vi "Configuração.vi"() -> ()   [LabVIEW 2018]
uses:
  Global_Telescopio.vi
panel:
  in  "URL do finals2000A.all:":string
  in  "Case Constant\n(See Context Help) 4":bool
  in  "Case Constant\n(See Context Help)":bool
  out "error out":errorcluster
  in  "Geral":T1(tab)=enum."Pos. Cúpula"
  in  "wheather timeout":bool
  in  "Tempo sem dados":dbl=120.0 caption="segundos" min=0.0
  in  "PressãoMax":dbl=1200.0 caption="mbar"
  in  "UmidadeMax":dbl=100.0 caption="%"
  in  "TemperaturaMax":dbl=30.0 caption="ºC"
  in  "PressãoMin":dbl=500.0 caption="mbar"
  in  "UmidadeMin":dbl caption="%"
  in  "TemperaturaMin":dbl caption="ºC"
  in  "Salvar valores":bool
  in  "Pressão atmosférica":dbl=880.0 caption="mbar"
  in  "Umidade":dbl=88.0 caption="%"
  in  "Temperatura":dbl=15.0 caption="ºC"
  in  "Default Met":bool
  in  "Memorizar Default Met":bool
  in  "Caminho Estação Meteorológica":string="V 1.0.0 arquivo obsoleto. Usado apenas PUB ZeroMQ."
  in  "Desloc_Min_Cúpula":i32=2 min=2
  in  "OffsetCupula":dbl=135.0 format="%#_11g"
  in  "Salvar dados cupula":bool
  in  "OffsetZ":dbl=-0.28 format="%#_11g"
  in  "OffsetY":dbl format="%#_11g"
  in  "OffsetX":dbl format="%#_11g"
  in  "DistEixos":dbl=-0.62 format="%#_11g"
  in  "RaioCup":dbl=3.2 format="%#_11g"
  in  "LATrad":dbl=5.889885056 format="%#_11g"
  out "Calagem DEC":string
  out "Calagem AH":string
  in  "LoadCalagem":bool
  in  "Instrumento":u16(ring) items=["Coude A+", "Coude B+", "ECass+", "Eucalyptus+", "Cam 1+", "Cam 2*", "Cam4 + IV*", "Polarimetro*", "Fortrap*", "Cam1 RF*", "Coude C+", "MUSICOS*", "+Já testado", "* nao config", "cam 1 s/rf", "cam1srf/luca+focali", "Coude A/luca", "ECass/luca", "Cam1+rf+luca", "MUSICOS+Luca", "Camiv+Luca", "Cam2+Luca", "Cam1+rf+luca+Ixon", "Cam1+rf+luca+Ikon", "CoudeTeste"]
  in  "Conf. Instrumentos":bool
  in  "Tabela Instrumentos":string[][](table)=[["Coude", "281.52", " 11.53", "S", "S", "0.462", "23.1", "23.1"], ["Cassegrain", "281.52", " 11.53", "S", "S", "0.462", "23.1", "23.1"], ["Eucalyptus", "281.52", " 11.53", "S", "S", "0.462", "23.1", "23.1"], ["Cam 1", "281.52", " 11.53", "S", "S", "0.462", "23.1", "23.1"], ["Cam 2", "281.52", " 11.53", "S", "S", "0.462", "23.1", "23.1"], ["Cam IV", "281.52", " 11.53", "S", "S", "0.462", "23.1", "23.1"], ["Polarimetro", "281.52", " 11.53", "S", "S", "0.462", "23.1", "23.1"], ["Fortrap", "281.52", " 11.53", "S", "S", "0.462", "23.1", "23.1"]]
  in  "CorrecaoMin":dbl=0.1
  in  "tel_sts1":bool[](array[boolean])=[TRUE, TRUE, TRUE, TRUE, FALSE, FALSE, TRUE]
  in  "Senha LEAF":string
  in  "Enable ventilador":bool=TRUE
  in  "habilita supervisao":bool
  in  "Tempo delay":i32=1
  in  "Limite Oeste":dbl=5.0 min=-12.0 max=12.0 step=0.1
  in  "Limite Leste":dbl=-4.5 min=-12.0 max=12.0 step=0.1
  out "DownloadWait":bool
  out "DownloadOK":bool caption="OK"
  in  "Download_Finals2000A.all":bool
  in  "Tempo Atualização All Sky":i32=1 min=1
  in  "Tempo Atualização Cam 3":i32=1 min=1
  in  "Tempo Atualização Cam 2":i32=1 min=1
  in  "Tempo Atualização Cam 1":i32=1 min=1
  in  "Tempo Atualização Cam 0":i32=1 min=1
  out "Ângulo Zenital":dbl format="%#.1f"
  out "Azimute":dbl format="%#.1f"
  in  "Tabela Proteção":string[][](table)=[["0", "360", "70", "60", "65"]]
  in  "Raio Máximo":dbl=5.0 min=0.0 max=90.0 step=0.1
  in  "Z_Max":dbl
  in  "Z_Libera":dbl
  in  "Z_Segurança":dbl
  in  "Hour Angle":string="00 00 0,00" caption="Dest AH"
  in  "Dest Dec":string="00 00 00,00"
  in  "SALVA CONFIG":bool
  out "DestDEC":dbl
  in  "DestCUP":i32
  out "DestAH":dbl
  in  "Caminho camera":string
  in  "Hora vent inicial":i32=1 min=0 max=86399 step=1 format="%<%H:%M:%S>t"
  in  "Hora vent final":i32=1 min=0 max=86399 step=1 format="%<%H:%M:%S>t"
  in  "ENGENHARIA":bool
  # "Configuração do Sistema"
  # "Caminho completo da Estação Meteorológica\nEx: http://200.131.64.185/clima/download.txt"
  # "Especifica o tempo para sinalizar que o TCSPD não está\nrecebendo os dados da estação meteorológica."
  # "Usar valores default se ocorrer a sinalização descrita acima."
  # "Valores Médios"
  # "Limite Mínimo"
  # "Limite Máximo"
  # "Quando \"Default Met\" for selecionado, sempre serão usados os valores médios (default) de temperatura, umidade e pressão atmosférica no cálculo da refração atmostérica e não os valores lidos da estação meteorológica, mesmo que estes sejam válidos e corretos."
  # "Se alguma leitura da estação meteorológica estiver fora dos limites acima, aquele valor será automaticamente substituído pelo seu valor médio."
  # "CONSTANTES DA CÚPULA"
  # "1,60m"
  # "IAG"
  # "5,889885056"
  # "5,889885056"
  # "7,525"
  # "3,20"
  # "-0,62"
  # "1,570"
  # "0,000"
  # "0,000"
  # "0,000"
  # "0,000"
  # "0,300"
  # "-0,28"
  # "136,0"
  # "-135,0"
  # "4"
  # "2"
  # "Valores default para o IAG (03/03/2011)"
  # "Ao precionar as Teclas de Captura\né necessário selecionar  a Região \nde interesse da imagem!"
  # "Selecione a Captrua\na ser posicionada"
  # "Seriais\nAuto Guider"
  # "Ângulo\nRotator"
  # "Ângulo\nNorte"
  # "Img.\nEsp."
  # "No\nCass."
  # "Escala\nPlaca"
  # "Calagem\nAH (\")"
  # "Calagem\nDEC (\")"
  # "Posição\nFoco"
  # "Escolha do Instrumento"
  # "Instrumento"
  # "Calagem"
  # "Carrega a calagem do telescópio com a calagem inicial do instrumento"
  # "CorrecaoMin: Valor em arcsec utilizado como limite para mover os\neixos AH e DEC nos processos de guiagem automática (auto-guider)\ne de offset do sistema de aquisição. Não será executado nenhum \nmovimento desses processos com deslocamento inferior a CorrecaoMin."
  # "Parâmetros PARK"
  # "Radianos"
  # "-->"
  # "Faixa do Azimute\n   De:              Ate:"
  # "Ângulo Zenital\n  Máx:       Segur.:       Libera:"
  # "-->"
  # "Raio da Calagem Local"
  # "Graus"
  # "Tempo de delay de comunicação"
  # "Arquivo finals2000A.all para precessão"
  # "Habilita Supervisão do Controlador"
  # "Horas"
  # "Horas"
  # "C:\\TCS\\ARQUIVOS\\finals2000A.all,  2,2Mb"
  # "Ventilador"
  # "Endereço da câmera"
  # "Usada na janela popup do Leaf e na\naba DOME que tem dupla função:abrir trapeira e habilitar movimento do telescópio com plataforma alta."
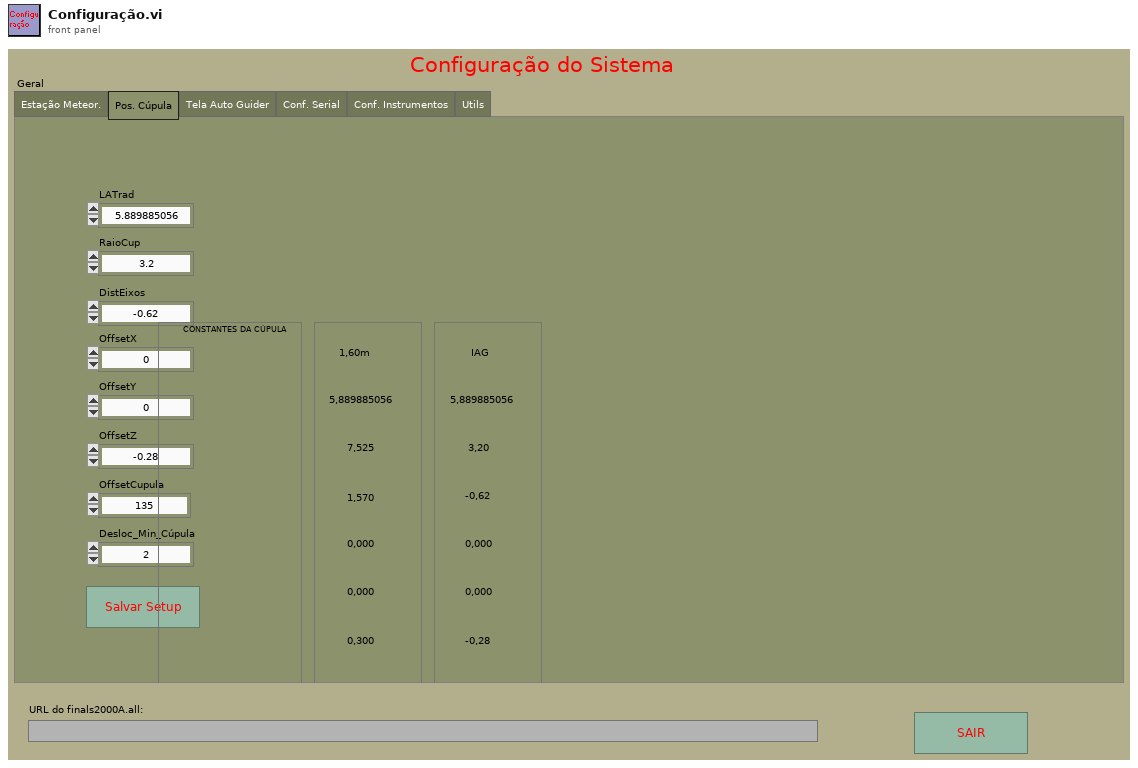
[diagram p1: front panel]
types:
  T1 = enum32{"Estação Meteor.", "Pos. Cúpula", "Tela Auto Guider", "Conf. Serial", "Conf. Instrumentos", "Utils"}
  T2 = cluster{"temperatura":dbl, "umidade":dbl, "pressao":dbl, "temperaturaMin":dbl, "umidadeMin":dbl, "pressaoMin":dbl, "temperaturaMax":dbl, "umidadeMax":dbl, "pressaoMax":dbl, "tempoSemDados":dbl}
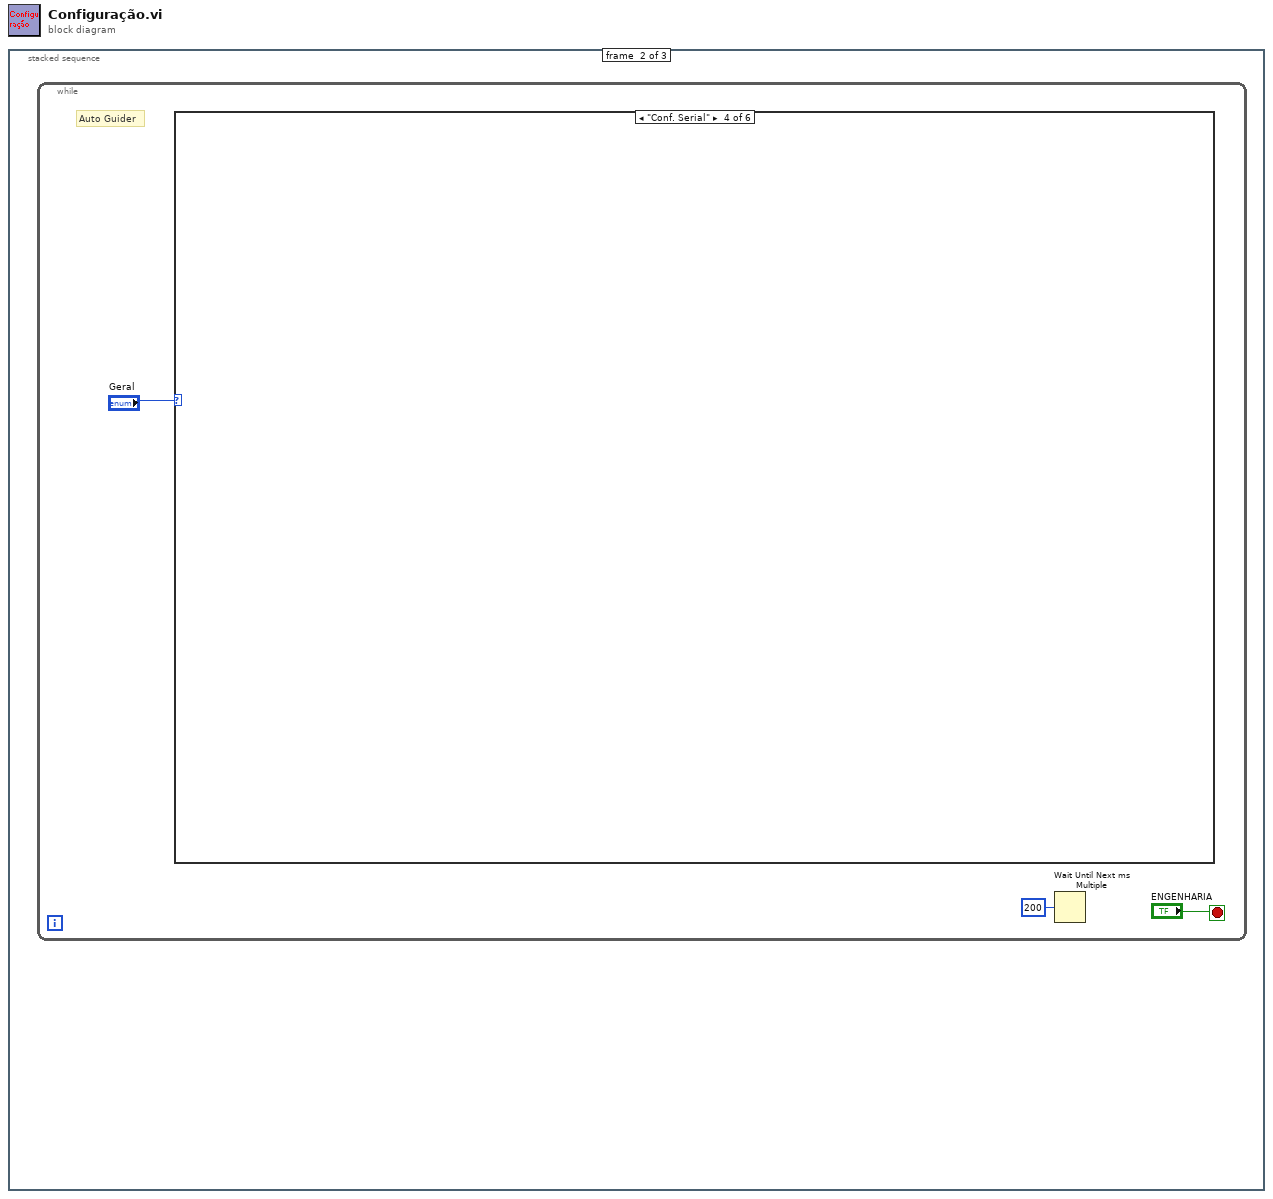
[diagram p0: block diagram]
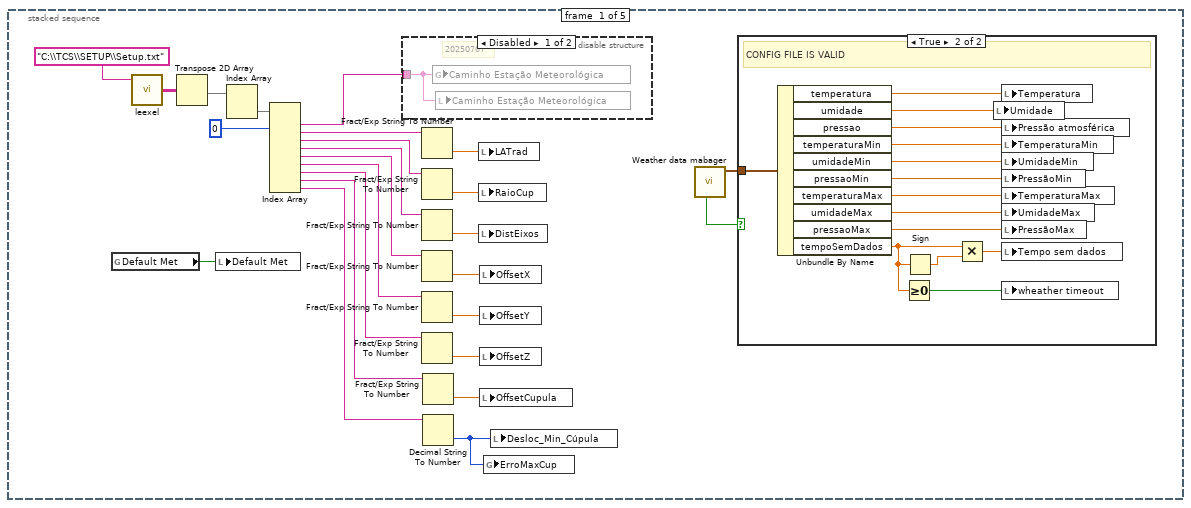
[diagram p3: hidden frame]
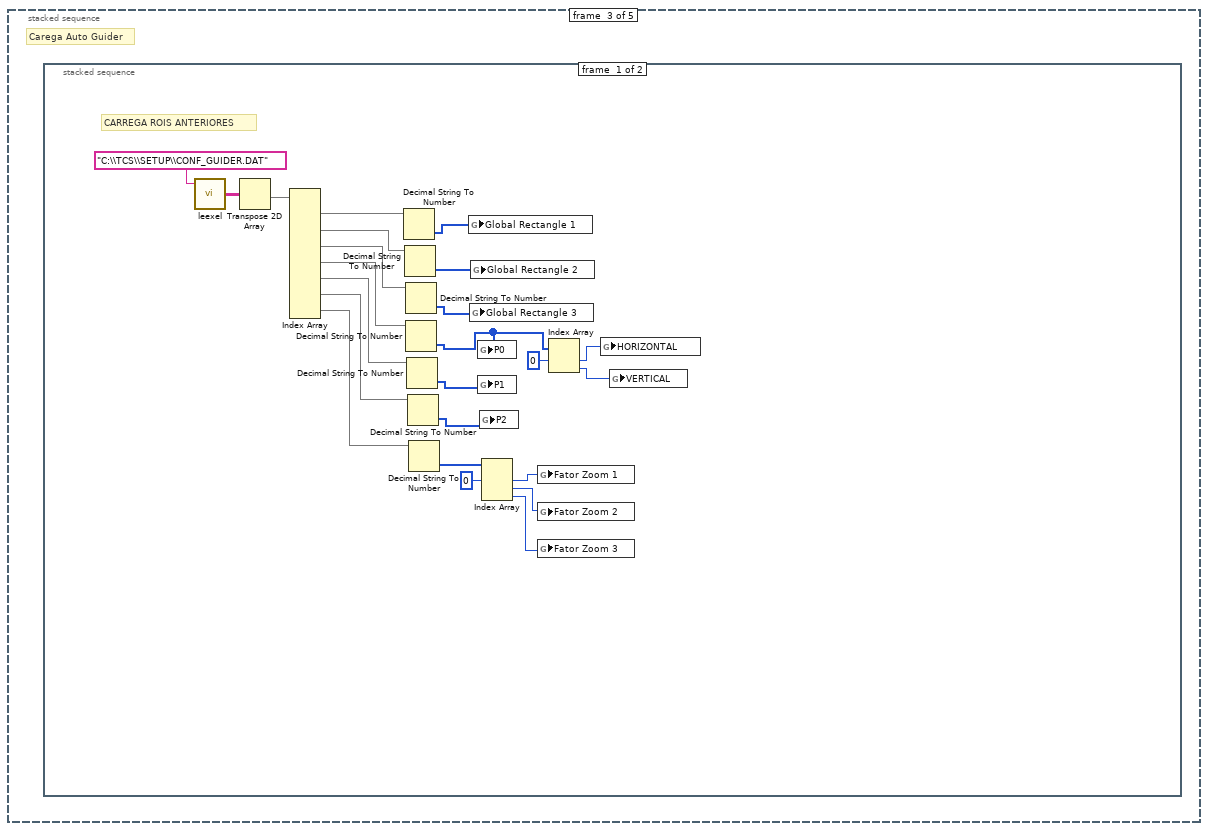
[diagram p6: hidden frame]
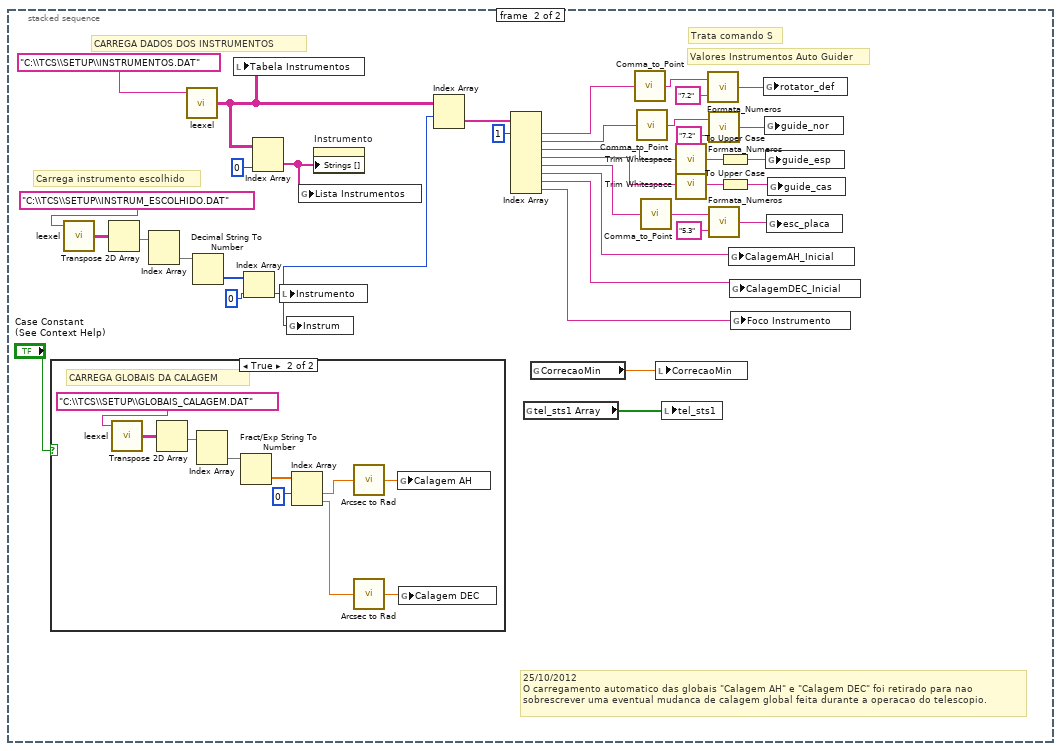
[diagram p7: hidden frame]
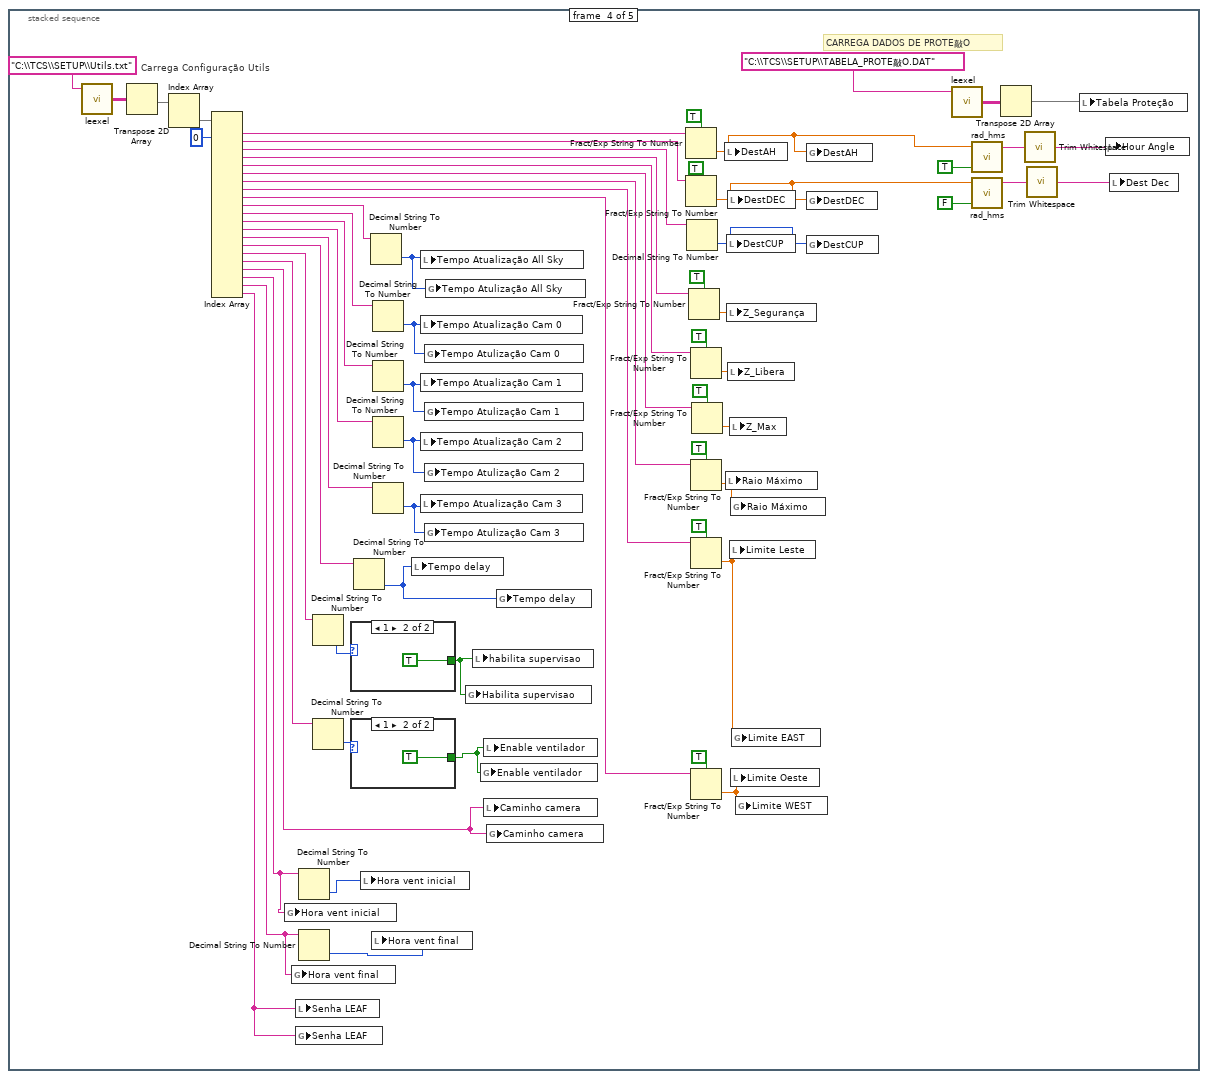
[diagram p9: hidden frame]
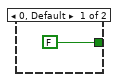
[diagram p10: hidden frame]
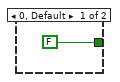
[diagram p11: hidden frame]
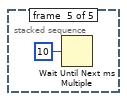
[diagram p12: hidden frame]
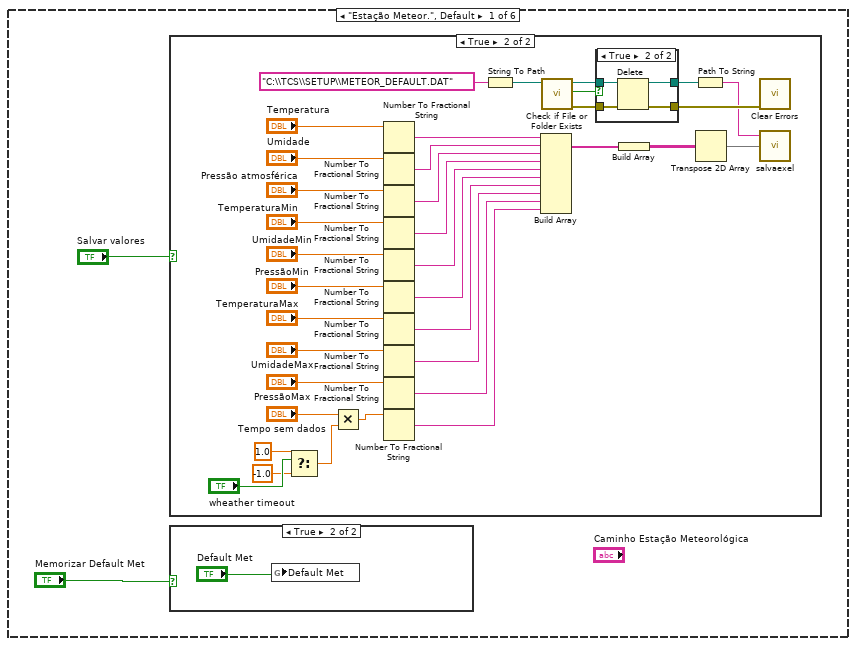
[diagram p13: hidden frame]
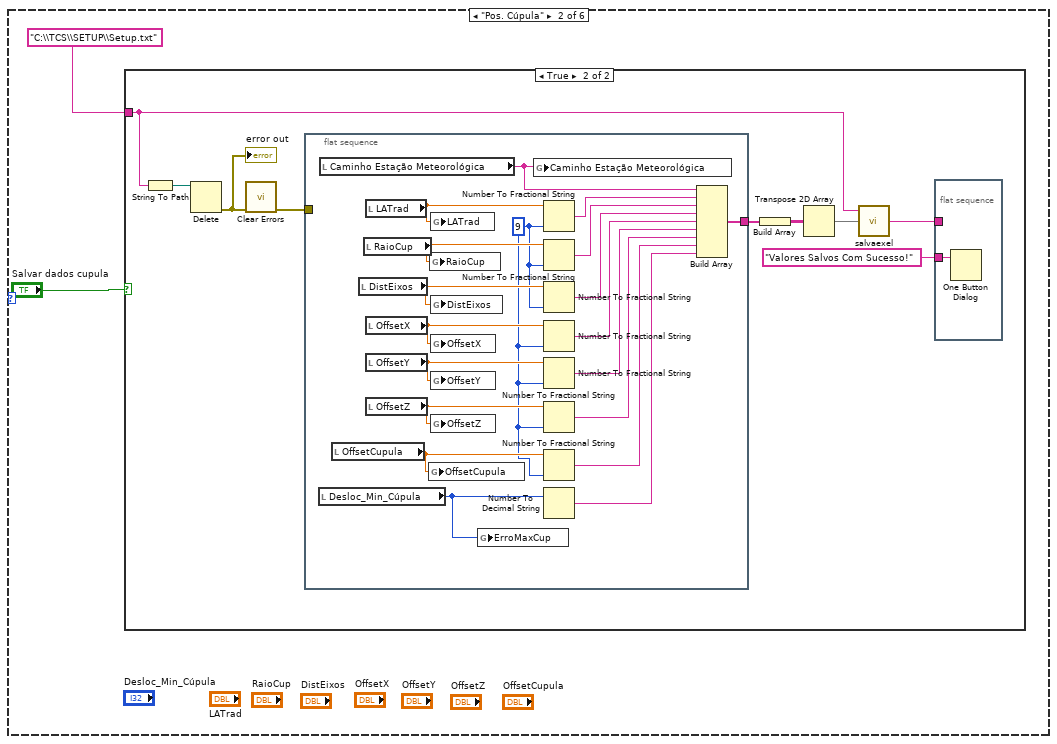
[diagram p17: hidden frame]
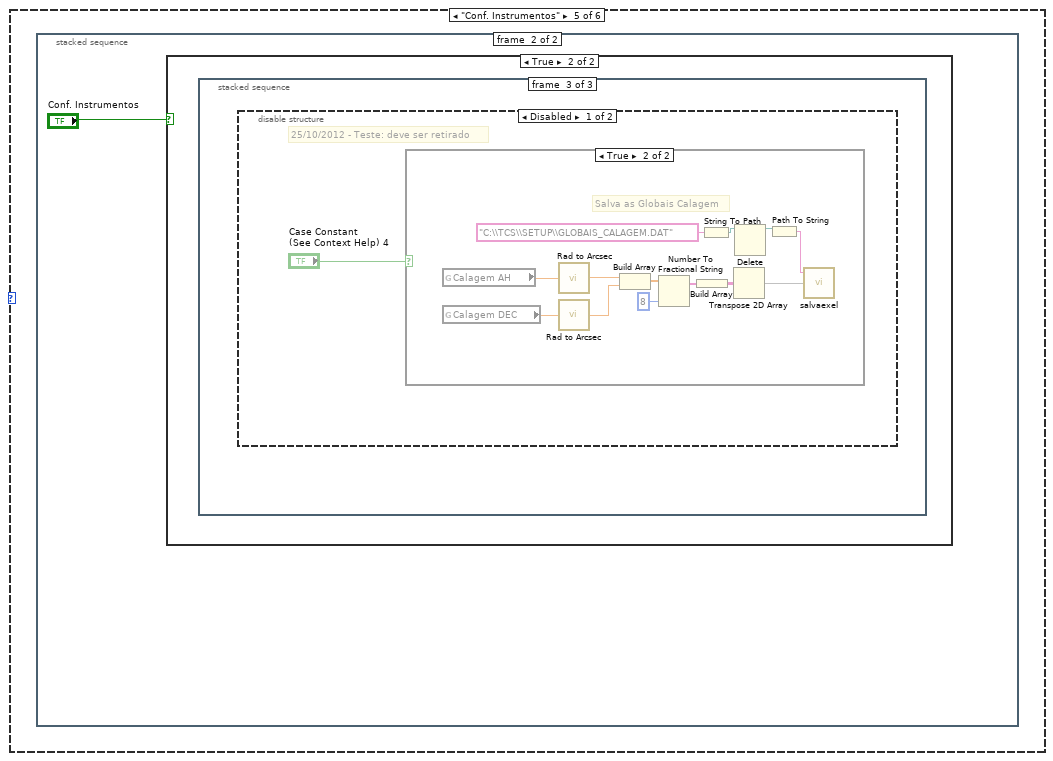
[diagram p20: hidden frame]
diagram:
  n1 = stacked-sequence {
    frame #0 {
      n2 = stacked-sequence {
        frame #0 {
          n3 = global read "Global_Telescopio.vi" "Default Met"() -> (w3:bool)
          n4 = call "leexel.vi"("path"="C:\\TCS\\SETUP\\Setup.txt") -> ("array 5"=w24:string[][])  [unwired: 4 in]
          n5 = Transpose 2D Array(2D array=w24) -> (transposed array=w23:string[][])
          n6 = local write "Default Met"(w3) -> ()
          n7 = Index Array(array=w23) -> (element=w22:string[])  [unwired: 2 in]
          n8 = Index Array(array=w22, index #1=0 ("index")) -> (element #1=w20:string, element #2=w18:string, element #3=w12:string, element #4=w11:string, element #5=w10:string, element #6=w9:string, element #7=w8:string, element #8=w6:string, element #9=w5:string)  [unwired: 8 in]
          n9 = disable-structure shown="Disabled" {
            disable-tunnel: w20 -> [w40 _]
            frame Disabled {
              # "20250707"
              n10 = global write "Global_Telescopio.vi" "Caminho Estação Meteorológica"(w40) -> ()
              n11 = local write "Caminho Estação Meteorológica"(w40) -> ()
            }
            frame Enabled {
            }
          }
          n12 = Fract/Exp String To Number(string=w18) -> (number=w19:dbl)  [unwired: 3 in, 1 out]
          n13 = Fract/Exp String To Number(string=w12) -> (number=w17:dbl)  [unwired: 3 in, 1 out]
          n14 = Fract/Exp String To Number(string=w11) -> (number=w16:dbl)  [unwired: 3 in, 1 out]
          n15 = Fract/Exp String To Number(string=w10) -> (number=w15:dbl)  [unwired: 3 in, 1 out]
          n16 = Fract/Exp String To Number(string=w9) -> (number=w14:dbl)  [unwired: 3 in, 1 out]
          n17 = Fract/Exp String To Number(string=w8) -> (number=w13:dbl)  [unwired: 3 in, 1 out]
          n18 = Fract/Exp String To Number(string=w6) -> (number=w7:dbl)  [unwired: 3 in, 1 out]
          n19 = Decimal String To Number(string=w5) -> (number=w4:i32)  [unwired: 2 in, 1 out]
          n20 = local write "LATrad"(w19) -> ()
          n21 = local write "RaioCup"(w17) -> ()
          n22 = local write "DistEixos"(w16) -> ()
          n23 = local write "OffsetX"(w15) -> ()
          n24 = local write "OffsetY"(w14) -> ()
          n25 = local write "OffsetZ"(w13) -> ()
          n26 = local write "OffsetCupula"(w7) -> ()
          n27 = global write "Global_Telescopio.vi" "ErroMaxCup"(w4) -> ()
          n28 = local write "Desloc_Min_Cúpula"(w4) -> ()
          n29 = call "Weather data mabager.vi"() -> ("weatherDefault"=w2:T2, "valid file"=w1:bool)  [unwired: 4 in, 6 out]
          n30 = case shown="True" w1 {
            tunnel: w2 -> [_ w39]
            frame False {
              # "INVALID CONFIG FILE - DOES NOT CHANGE DEFAULT CONTROL VALUES"
            }
            frame True {
              # "CONFIG FILE IS VALID"
              n31 = Unbundle By Name(w39) -> ("temperatura"=w38:dbl, "umidade"=w37:dbl, "pressao"=w36:dbl, "temperaturaMin"=w35:dbl, "umidadeMin"=w34:dbl, "pressaoMin"=w33:dbl, "temperaturaMax"=w32:dbl, "umidadeMax"=w31:dbl, "pressaoMax"=w30:dbl, "tempoSemDados"=w28:dbl)
              n32 = Greater Or Equal To 0?(x=w28) -> (x >= 0?=w29:bool)
              n33 = Sign(1:w28) -> (0:w27:dbl)
              n34 = Multiply(x=w28, y=w27) -> (x*y=w26:dbl)
              n35 = local write "Umidade"(w37) -> ()
              n36 = local write "Temperatura"(w38) -> ()
              n37 = local write "Pressão atmosférica"(w36) -> ()
              n38 = local write "TemperaturaMin"(w35) -> ()
              n39 = local write "UmidadeMin"(w34) -> ()
              n40 = local write "PressãoMin"(w33) -> ()
              n41 = local write "TemperaturaMax"(w32) -> ()
              n42 = local write "UmidadeMax"(w31) -> ()
              n43 = local write "PressãoMax"(w30) -> ()
              n44 = local write "Tempo sem dados"(w26) -> ()
              n45 = local write "wheather timeout"(w29) -> ()
            }
          }
        }
        frame #1 {
        }
        frame #2 {
          # "Carega Auto Guider"
          n46 = stacked-sequence {
            frame #0 {
              # "CARREGA ROIS ANTERIORES"
              n47 = call "leexel.vi"("path"="C:\\TCS\\SETUP\\CONF_GUIDER.DAT") -> ("array 5"=w63:string[][])  [unwired: 4 in]
              n48 = Transpose 2D Array(2D array=w63) -> (transposed array=w62:string[][])
              n49 = Index Array(array=w62) -> (element #1=w61:string[], element #2=w60:string[], element #3=w59:string[], element #4=w58:string[], element #5=w57:string[], element #6=w56:string[], element #7=w44:string[])  [unwired: 14 in]
              n50 = Decimal String To Number(string=w61) -> (number=w47:i32[])  [unwired: 2 in, 1 out]
              n51 = Decimal String To Number(string=w60) -> (number=w48:i32[])  [unwired: 2 in, 1 out]
              n52 = Decimal String To Number(string=w59) -> (number=w49:i32[])  [unwired: 2 in, 1 out]
              n53 = Decimal String To Number(string=w58) -> (number=w52:i32[])  [unwired: 2 in, 1 out]
              n54 = Decimal String To Number(string=w57) -> (number=w51:i32[])  [unwired: 2 in, 1 out]
              n55 = Decimal String To Number(string=w56) -> (number=w50:i32[])  [unwired: 2 in, 1 out]
              n56 = Decimal String To Number(string=w44) -> (number=w43:i32[])  [unwired: 2 in, 1 out]
              n57 = global write "Global_Telescopio.vi" "Global Rectangle 1"(w47) -> ()
              n58 = global write "Global_Telescopio.vi" "Global Rectangle 3"(w49) -> ()
              n59 = global write "Global_Telescopio.vi" "Global Rectangle 2"(w48) -> ()
              n60 = global write "Global_Telescopio.vi" "P0"(w52) -> ()
              n61 = global write "Global_Telescopio.vi" "P1"(w51) -> ()
              n62 = global write "Global_Telescopio.vi" "P2"(w50) -> ()
              n63 = Index Array(array=w43, index #1=0 ("index")) -> (element #1=w45:i32, element #2=w42:i32, element #3=w41:i32)  [unwired: 2 in]
              n64 = global write "Global_Telescopio.vi" "Fator Zoom 1"(w45) -> ()
              n65 = global write "Global_Telescopio.vi" "Fator Zoom 2"(w42) -> ()
              n66 = global write "Global_Telescopio.vi" "Fator Zoom 3"(w41) -> ()
              n67 = Index Array(array=w52, index #1=0 ("index")) -> (element #1=w54:i32, element #2=w53:i32)  [unwired: 1 in]
              n68 = global write "Global_Telescopio.vi" "HORIZONTAL"(w54) -> ()
              n69 = global write "Global_Telescopio.vi" "VERTICAL"(w53) -> ()
            }
            frame #1 {
              # "25/10/2012\nO carregamento automatico das globais \"Calagem AH\" e \"Calagem DEC\" foi retirado para nao \nsobrescrever uma eventual mudanca de calagem global feita durante a operacao do telescopio."
              # "Trata comando S"
              # "Valores Instrumentos Auto Guider"
              # "Carrega instrumento escolhido"
              # "CARREGA DADOS DOS INSTRUMENTOS"
              n70 = case shown="True" "Case Constant\n(See Context Help)" {
                frame False {
                }
                frame True {
                  # "CARREGA GLOBAIS DA CALAGEM"
                  n71 = call "leexel.vi"("path"="C:\\TCS\\SETUP\\GLOBAIS_CALAGEM.DAT") -> ("array 5"=w108:string[][])  [unwired: 4 in]
                  n72 = Transpose 2D Array(2D array=w108) -> (transposed array=w109:string[][])
                  n73 = Index Array(array=w109) -> (element=w107:string[])  [unwired: 2 in]
                  n74 = Fract/Exp String To Number(string=w107) -> (number=w111:dbl[])  [unwired: 3 in, 1 out]
                  n75 = Index Array(array=w111, index #1=0 ("index")) -> (element #1=w105:dbl, element #2=w104:dbl)  [unwired: 1 in]
                  n76 = call "Arcsec to Rad.vi"("Arcsec"=w105) -> ("rad"=w103:dbl)
                  n77 = call "Arcsec to Rad.vi"("Arcsec"=w104) -> ("rad"=w102:dbl)
                  n78 = global write "Global_Telescopio.vi" "Calagem AH"(w103) -> ()
                  n79 = global write "Global_Telescopio.vi" "Calagem DEC"(w102) -> ()
                }
              }
              n80 = call "leexel.vi"("path"="C:\\TCS\\SETUP\\INSTRUM_ESCOLHIDO.DAT") -> ("array 5"=w97:string[][])  [unwired: 4 in]
              n81 = Transpose 2D Array(2D array=w97) -> (transposed array=w96:string[][])
              n82 = Index Array(array=w96) -> (element=w98:string[])  [unwired: 2 in]
              n83 = call "leexel.vi"("path"="C:\\TCS\\SETUP\\INSTRUMENTOS.DAT") -> ("array 5"=w93:string[][])  [unwired: 4 in]
              n84 = Decimal String To Number(string=w98) -> (number=w94:i32[])  [unwired: 2 in, 1 out]
              n85 = local write "Tabela Instrumentos"(w93) -> ()
              n86 = Index Array(array=w94, index=0) -> (element=w85:i32)
              n87 = Index Array(array=w93, index (col)=0 ("disabled index (col)")) -> (element=w86:string[])  [unwired: 1 in]
              n88 = local write "Instrumento"(w85) -> ()
              n89 = global write "Global_Telescopio.vi" "Instrum"(w85) -> ()
              n90 = global write "Global_Telescopio.vi" "Lista Instrumentos"(w86) -> ()
              n91 = property on="Instrumento" class="Ring (strict)"("Strings []"=w86) -> ()  [unwired: 2 in, 2 out]
              n92 = Index Array(array=w93, index (row)=w85) -> (element=w91:string[])  [unwired: 1 in]
              n93 = Index Array(array=w91, index #1=1 ("index")) -> (element #1=w81:string, element #2=w77:string, element #3=w74:string, element #4=w71:string, element #5=w67:string, element #6=w88:string, element #7=w87:string, element #8=w66:string)  [unwired: 7 in]
              n94 = global read "Global_Telescopio.vi" "tel_sts1 Array"() -> (w89:bool[])
              n95 = global read "Global_Telescopio.vi" "CorrecaoMin"() -> (w90:dbl)
              n96 = call "Comma_to_Point.vi"("Lat_A"=w81) -> ("Saída"=w82:string)
              n97 = call "Comma_to_Point.vi"("Lat_A"=w77) -> ("Saída"=w78:string)
              n98 = call "Comma_to_Point.vi"("Lat_A"=w67) -> ("Saída"=w68:string)
              n99 = local write "CorrecaoMin"(w90) -> ()
              n100 = local write "tel_sts1"(w89) -> ()
              n101 = call <vilib>:"Trim Whitespace.vi"("string"=w74) -> ("trimmed string"=w76:string)  [unwired: 1 in]
              n102 = call <vilib>:"Trim Whitespace.vi"("string"=w71) -> ("trimmed string"=w73:string)  [unwired: 1 in]
              n103 = call "Formata_Numeros.vi"("Formato ex-> 7.2"="7.2", "Valor num"=w82) -> ("resulting string"=w83:string)
              n104 = call "Formata_Numeros.vi"("Formato ex-> 7.2"="7.2", "Valor num"=w78) -> ("resulting string"=w79:string)
              n105 = call "Formata_Numeros.vi"("Formato ex-> 7.2"="5.3", "Valor num"=w68) -> ("resulting string"=w69:string)
              n106 = To Upper Case(1:w76) -> (0:w75:string)
              n107 = To Upper Case(1:w73) -> (0:w72:string)
              n108 = global write "Global_Telescopio.vi" "CalagemAH_Inicial"(w88) -> ()
              n109 = global write "Global_Telescopio.vi" "CalagemDEC_Inicial"(w87) -> ()
              n110 = global write "Global_Telescopio.vi" "Foco Instrumento"(w66) -> ()
              n111 = global write "Global_Telescopio.vi" "rotator_def"(w83) -> ()
              n112 = global write "Global_Telescopio.vi" "guide_nor"(w79) -> ()
              n113 = global write "Global_Telescopio.vi" "guide_esp"(w75) -> ()
              n114 = global write "Global_Telescopio.vi" "esc_placa"(w69) -> ()
              n115 = global write "Global_Telescopio.vi" "guide_cas"(w72) -> ()
            }
          }
        }
        frame #3 {
          # "CARREGA DADOS DE PROTE敲O"
          # "Carrega Configuração Utils"
          n116 = call "leexel.vi"("path"="C:\\TCS\\SETUP\\Utils.txt") -> ("array 5"=w174:string[][])  [unwired: 4 in]
          n117 = Transpose 2D Array(2D array=w174) -> (transposed array=w173:string[][])
          n118 = Index Array(array=w173) -> (element=w172:string[])  [unwired: 2 in]
          n119 = Index Array(array=w172, index #1=0 ("index")) -> (element #1=w170:string, element #2=w169:string, element #3=w168:string, element #4=w153:string, element #5=w152:string, element #6=w151:string, element #7=w145:string, element #8=w127:string, element #9=w126:string, element #10=w132:string, element #11=w133:string, element #12=w134:string, element #13=w135:string, element #14=w136:string, element #15=w125:string, element #16=w124:string, element #17=w117:string, element #18=w118:string, element #19=w113:string, element #20=w114:string, element #21=w112:string)  [unwired: 20 in]
          n120 = global write "Global_Telescopio.vi" "Hora vent inicial"(w113) -> ()
          n121 = global write "Global_Telescopio.vi" "Hora vent final"(w114) -> ()
          n122 = local write "Senha LEAF"(w112) -> ()
          n123 = global write "Global_Telescopio.vi" "Senha LEAF"(w112) -> ()
          n124 = Decimal String To Number(string=w113) -> (number=w116:i32)  [unwired: 2 in, 1 out]
          n125 = Decimal String To Number(string=w114) -> (number=w115:i32)  [unwired: 2 in, 1 out]
          n126 = Decimal String To Number(string=w124) -> (number=w123:i32)  [unwired: 2 in, 1 out]
          n127 = Decimal String To Number(string=w117) -> (number=w120:i32)  [unwired: 2 in, 1 out]
          n128 = case shown="1" w123 {
            tunnel: [FALSE TRUE] -> w122
            frame 0, Default {
            }
            frame 1 {
            }
          }
          n129 = case shown="1" w120 {
            tunnel: [FALSE TRUE] -> w119
            frame 0, Default {
            }
            frame 1 {
            }
          }
          n130 = Decimal String To Number(string=w125) -> (number=w121:i32)  [unwired: 2 in, 1 out]
          n131 = local write "Hora vent inicial"(w116) -> ()
          n132 = Decimal String To Number(string=w132) -> (number=w141:i32)  [unwired: 2 in, 1 out]
          n133 = local write "Hora vent final"(w115) -> ()
          n134 = Decimal String To Number(string=w133) -> (number=w140:i32)  [unwired: 2 in, 1 out]
          n135 = Decimal String To Number(string=w134) -> (number=w139:i32)  [unwired: 2 in, 1 out]
          n136 = Decimal String To Number(string=w135) -> (number=w138:i32)  [unwired: 2 in, 1 out]
          n137 = Decimal String To Number(string=w136) -> (number=w137:i32)  [unwired: 2 in, 1 out]
          n138 = local write "Tempo delay"(w121) -> ()
          n139 = local write "Tempo Atualização All Sky"(w141) -> ()
          n140 = local write "Tempo Atualização Cam 0"(w140) -> ()
          n141 = local write "Tempo Atualização Cam 1"(w139) -> ()
          n142 = local write "Tempo Atualização Cam 2"(w138) -> ()
          n143 = local write "Tempo Atualização Cam 3"(w137) -> ()
          n144 = global write "Global_Telescopio.vi" "Tempo Atulização Cam 0"(w140) -> ()
          n145 = global write "Global_Telescopio.vi" "Tempo Atulização Cam 1"(w139) -> ()
          n146 = global write "Global_Telescopio.vi" "Tempo Atulização Cam 2"(w138) -> ()
          n147 = global write "Global_Telescopio.vi" "Tempo Atulização Cam 3"(w137) -> ()
          n148 = global write "Global_Telescopio.vi" "Tempo Atulização All Sky"(w141) -> ()
          n149 = global write "Global_Telescopio.vi" "Habilita supervisao"(w122) -> ()
          n150 = local write "habilita supervisao"(w122) -> ()
          n151 = global write "Global_Telescopio.vi" "Enable ventilador"(w119) -> ()
          n152 = local write "Enable ventilador"(w119) -> ()
          n153 = local write "Caminho camera"(w118) -> ()
          n154 = global write "Global_Telescopio.vi" "Caminho camera"(w118) -> ()
          n155 = global write "Global_Telescopio.vi" "Tempo delay"(w121) -> ()
          n156 = Fract/Exp String To Number(use system decimal point (T)=TRUE, string=w170) -> (number=w164:dbl)  [unwired: 2 in, 1 out]
          n157 = Fract/Exp String To Number(use system decimal point (T)=TRUE, string=w169) -> (number=w163:dbl)  [unwired: 2 in, 1 out]
          n158 = Decimal String To Number(string=w168) -> (number=w167:i32)  [unwired: 2 in, 1 out]
          n159 = Fract/Exp String To Number(use system decimal point (T)=TRUE, string=w153) -> (number=w150:dbl)  [unwired: 2 in, 1 out]
          n160 = Fract/Exp String To Number(use system decimal point (T)=TRUE, string=w152) -> (number=w149:dbl)  [unwired: 2 in, 1 out]
          n161 = Fract/Exp String To Number(use system decimal point (T)=TRUE, string=w145) -> (number=w146:dbl)  [unwired: 2 in, 1 out]
          n162 = Fract/Exp String To Number(use system decimal point (T)=TRUE, string=w127) -> (number=w128:dbl)  [unwired: 2 in, 1 out]
          n163 = Fract/Exp String To Number(use system decimal point (T)=TRUE, string=w126) -> (number=w129:dbl)  [unwired: 2 in, 1 out]
          n164 = Fract/Exp String To Number(use system decimal point (T)=TRUE, string=w151) -> (number=w148:dbl)  [unwired: 2 in, 1 out]
          n165 = local write "DestAH"(w164) -> ()
          n166 = local write "Raio Máximo"(w146) -> ()
          n167 = local write "DestCUP"(w167) -> ()
          n168 = local write "Z_Segurança"(w150) -> ()
          n169 = local write "DestDEC"(w163) -> ()
          n170 = local write "Z_Libera"(w149) -> ()
          n171 = local write "Z_Max"(w148) -> ()
          n172 = local write "Limite Leste"(w128) -> ()
          n173 = global write "Global_Telescopio.vi" "Raio Máximo"(w146) -> ()
          n174 = local write "Limite Oeste"(w129) -> ()
          n175 = global write "Global_Telescopio.vi" "Limite EAST"(w128) -> ()
          n176 = global write "Global_Telescopio.vi" "Limite WEST"(w129) -> ()
          n177 = global write "Global_Telescopio.vi" "DestAH"(w164) -> ()
          n178 = global write "Global_Telescopio.vi" "DestDEC"(w163) -> ()
          n179 = global write "Global_Telescopio.vi" "DestCUP"(w167) -> ()
          n180 = call "leexel.vi"("path"="C:\\TCS\\SETUP\\TABELA_PROTE敲O.DAT") -> ("array 5"=w143:string[][])  [unwired: 4 in]
          n181 = call "rad_hms.vi"("TRUE=HORA\nFALSE=GRAU"=TRUE, "Radiano"=w164) -> ("Hora/Graus Texto Decimal"=w158:string)  [unwired: 3 in]
          n182 = call "rad_hms.vi"("TRUE=HORA\nFALSE=GRAU"=FALSE, "Radiano"=w163) -> ("Hora/Graus Texto Decimal"=w157:string)  [unwired: 3 in]
          n183 = Transpose 2D Array(2D array=w143) -> (transposed array=w142:string[][])
          n184 = call <vilib>:"Trim Whitespace.vi"("string"=w158) -> ("trimmed string"=w159:string)  [unwired: 1 in]
          n185 = call <vilib>:"Trim Whitespace.vi"("string"=w157) -> ("trimmed string"=w160:string)  [unwired: 1 in]
          n186 = local write "Tabela Proteção"(w142) -> ()
          n187 = local write "Hour Angle"(w159) -> ()
          n188 = local write "Dest Dec"(w160) -> ()
        }
        frame #4 {
          n189 = Wait Until Next ms Multiple(millisecond multiple=u32 10) -> ()  [unwired: 1 out]
        }
      }
    }
    frame #1 {
      n190 = while {
        stop <- "ENGENHARIA" stop-if-true
        # "Auto Guider"
        n191 = case shown="\"Conf. Serial\"" "Geral" {
          frame "Estação Meteor.", Default {
            n192 = case shown="True" "Salvar valores" {
              frame False {
              }
              frame True {
                n193 = Select(t=1.0, s="wheather timeout", f=-1.0 ("t")) -> (s? t:f=w189:dbl)
                n194 = Multiply(x="Tempo sem dados", y=w189) -> (x*y=w191:dbl)
                n195 = Number To Fractional String(number="Temperatura") -> (F-format string=w220:string)  [unwired: 3 in]
                n196 = Number To Fractional String(number="Umidade") -> (F-format string=w219:string)  [unwired: 3 in]
                n197 = Number To Fractional String(number="Pressão atmosférica") -> (F-format string=w218:string)  [unwired: 3 in]
                n198 = Number To Fractional String(number="TemperaturaMin") -> (F-format string=w198:string)  [unwired: 3 in]
                n199 = Number To Fractional String(number="UmidadeMin") -> (F-format string=w197:string)  [unwired: 3 in]
                n200 = Number To Fractional String(number="PressãoMin") -> (F-format string=w196:string)  [unwired: 3 in]
                n201 = Number To Fractional String(number="TemperaturaMax") -> (F-format string=w195:string)  [unwired: 3 in]
                n202 = Number To Fractional String(number="UmidadeMax") -> (F-format string=w194:string)  [unwired: 3 in]
                n203 = Number To Fractional String(number="PressãoMax") -> (F-format string=w193:string)  [unwired: 3 in]
                n204 = Number To Fractional String(number=w191) -> (F-format string=w192:string)  [unwired: 3 in]
                n205 = String To Path(string="C:\\TCS\\SETUP\\METEOR_DEFAULT.DAT") -> (path=w211:path)
                n206 = Build Array(w220, w219, w218, w198, w197, w196, w195, w194, w193, w192) -> (w214:string[])
                n207 = call <vilib>:"Check if File or Folder Exists.vi"("path"=w211) -> ("error out"=w209:errorcluster, "file or folder exists?"=w208:bool, "dup path"=w210:path)  [unwired: 8 in]
                n208 = case shown="True" w208 {
                  tunnel: [w222 w227] -> w212
                  tunnel: w210 -> [w223 w226]
                  tunnel: w209 -> [w222 w225]
                  tunnel: [w223 w224] -> w207
                  frame False {
                  }
                  frame True {
                    n209 = Delete(path (use dialog)=w226, error in=w225) -> (deleted path=w224:path, error out=w227:errorcluster)  [unwired: 3 in, 1 out]
                  }
                }
                n210 = Build Array(w214) -> (w213:string[][])
                n211 = Path To String(path=w207) -> (string=w205:string)
                n212 = Transpose 2D Array(2D array=w213) -> (transposed array=w221:string[][])
                n213 = call <vilib>:"Clear Errors.vi"("error in (no error)"=w212) -> ()  [unwired: 5 in, 2 out]
                n214 = call "salvaexel.vi"("appended array"=w221, "file name p/ exell"=w205) -> ()  [unwired: 1 in, 1 out]
              }
            }
            n215 = case shown="True" "Memorizar Default Met" {
              frame False {
              }
              frame True {
                n216 = global write "Global_Telescopio.vi" "Default Met"("Default Met") -> ()
              }
            }
          }
          frame "Pos. Cúpula" {
            n217 = case shown="True" "Salvar dados cupula" {
              tunnel: "C:\\TCS\\SETUP\\Setup.txt" -> [_ w233]
              frame False {
              }
              frame True {
                n218 = String To Path(string=w233) -> (path=w239:path)
                n219 = Delete(path (use dialog)=w239) -> (error out=w238:errorcluster)  [unwired: 4 in, 2 out]
                "error out" <- w238
                n220 = call <vilib>:"Clear Errors.vi"("error in (no error)"=w238) -> ("error out"=w237:errorcluster)  [unwired: 5 in, 1 out]
                n221 = flat-sequence {
                  tunnel: w237 -> [_]
                  tunnel: [w242] -> w234
                  frame #0 {
                    w243 = i16 9 ("precision (6)")
                    n222 = local read "Desloc_Min_Cúpula"() -> (w251:i32)
                    n223 = local read "Caminho Estação Meteorológica"() -> (w241:string)
                    n224 = local read "OffsetCupula"() -> (w244:dbl)
                    n225 = local read "DistEixos"() -> (w248:dbl)
                    n226 = local read "RaioCup"() -> (w249:dbl)
                    n227 = local read "LATrad"() -> (w250:dbl)
                    n228 = local read "OffsetX"() -> (w247:dbl)
                    n229 = local read "OffsetY"() -> (w246:dbl)
                    n230 = local read "OffsetZ"() -> (w245:dbl)
                    n231 = global write "Global_Telescopio.vi" "OffsetCupula"(w244) -> ()
                    n232 = global write "Global_Telescopio.vi" "RaioCup"(w249) -> ()
                    n233 = global write "Global_Telescopio.vi" "LATrad"(w250) -> ()
                    n234 = global write "Global_Telescopio.vi" "DistEixos"(w248) -> ()
                    n235 = global write "Global_Telescopio.vi" "OffsetX"(w247) -> ()
                    n236 = global write "Global_Telescopio.vi" "OffsetY"(w246) -> ()
                    n237 = global write "Global_Telescopio.vi" "OffsetZ"(w245) -> ()
                    n238 = global write "Global_Telescopio.vi" "ErroMaxCup"(w251) -> ()
                    n239 = global write "Global_Telescopio.vi" "Caminho Estação Meteorológica"(w241) -> ()
                    n240 = Number To Fractional String(number=w250, precision (6)=w243) -> (F-format string=w259:string)  [unwired: 2 in]
                    n241 = Number To Fractional String(number=w249, precision (6)=w243) -> (F-format string=w258:string)  [unwired: 2 in]
                    n242 = Number To Fractional String(number=w248, precision (6)=w243) -> (F-format string=w257:string)  [unwired: 2 in]
                    n243 = Number To Fractional String(number=w247, precision (6)=w243) -> (F-format string=w256:string)  [unwired: 2 in]
                    n244 = Number To Fractional String(number=w246, precision (6)=w243) -> (F-format string=w255:string)  [unwired: 2 in]
                    n245 = Number To Fractional String(number=w245, precision (6)=w243) -> (F-format string=w254:string)  [unwired: 2 in]
                    n246 = Number To Fractional String(number=w244, precision (6)=w243) -> (F-format string=w253:string)  [unwired: 2 in]
                    n247 = Number To Decimal String(number=w251) -> (decimal integer string=w252:string)  [unwired: 1 in]
                    n248 = Build Array(w241, w259, w258, w257, w256, w255, w254, w253, w252) -> (w242:string[])
                  }
                }
                n249 = Build Array(w234) -> (w236:string[][])
                n250 = Transpose 2D Array(2D array=w236) -> (transposed array=w235:string[][])
                n251 = call "salvaexel.vi"("appended array"=w235, "file name p/ exell"=w233) -> ("spreadsheet string"=w231:string)  [unwired: 1 in]
                n252 = flat-sequence {
                  tunnel: "Valores Salvos Com Sucesso!" ("message") -> [w240]
                  tunnel: w231 -> [_]
                  frame #0 {
                    n253 = One Button Dialog(message=w240) -> ()  [unwired: 1 in, 1 out]
                  }
                }
              }
            }
          }
          frame "Tela Auto Guider" {
          }
          frame "Conf. Serial" {
          }
          frame "Conf. Instrumentos" {
            n254 = stacked-sequence {
              frame #0 {
                w262 = i16 1 ("precision (6)")
                n255 = global read "Global_Telescopio.vi" "Calagem AH"() -> (w263:dbl)
                n256 = global read "Global_Telescopio.vi" "Calagem DEC"() -> (w266:dbl)
                n257 = local read "Tabela Instrumentos"() -> (w270:string[][])
                n258 = call "Rad to Arcsec.vi"("Radiano"=w266) -> ("Arcsec"=w265:dbl)
                n259 = call "Rad to Arcsec.vi"("Radiano"=w263) -> ("Arcsec"=w264:dbl)
                n260 = Number To Fractional String(number=w265, precision (6)=w262) -> (F-format string=→"Calagem DEC":string)  [unwired: 2 in]
                n261 = Number To Fractional String(number=w264, precision (6)=w262) -> (F-format string=→"Calagem AH":string)  [unwired: 2 in]
                n262 = Index Array(array=w270, index (col)=0 ("disabled index (col)")) -> (element=w268:string[])  [unwired: 1 in]
                n263 = property on="Instrumento" class="Ring (strict)"("Strings []"=w268) -> ()  [unwired: 2 in, 2 out]
                n264 = case shown="True" "LoadCalagem" {
                  selector: "LoadCalagem" -> [_ w273]
                  frame False {
                  }
                  frame True {
                    # "Faz a Calagem do telescópio igual à calagem inicial do instrumento"
                    n265 = global read "Global_Telescopio.vi" "CalagemDEC_Inicial"() -> (w275:string)
                    n266 = global read "Global_Telescopio.vi" "CalagemAH_Inicial"() -> (w279:string)
                    n267 = global write "Global_Telescopio.vi" "Flag-Rotator"(w273) -> ()
                    n268 = Fract/Exp String To Number(string=w279) -> (number=w278:dbl)  [unwired: 3 in, 1 out]
                    n269 = Fract/Exp String To Number(string=w275) -> (number=w276:dbl)  [unwired: 3 in, 1 out]
                    n270 = call "Arcsec to Rad.vi"("Arcsec"=w278) -> ("rad"=w277:dbl)
                    n271 = call "Arcsec to Rad.vi"("Arcsec"=w276) -> ("rad"=w274:dbl)
                    n272 = global write "Global_Telescopio.vi" "Calagem AH"(w277) -> ()
                    n273 = global write "Global_Telescopio.vi" "Calagem DEC"(w274) -> ()
                  }
                }
                n274 = global write "Global_Telescopio.vi" "CorrecaoMin"("CorrecaoMin") -> ()
                n275 = global write "Global_Telescopio.vi" "tel_sts1 Array"("tel_sts1") -> ()
              }
              frame #1 {
                n276 = case shown="True" "Conf. Instrumentos" {
                  frame False {
                  }
                  frame True {
                    n277 = stacked-sequence {
                      frame #0 {
                        n278 = local read "Instrumento"() -> (w281:u16)
                        n279 = local read "Tabela Instrumentos"() -> (w290:string[][])
                        n280 = Build Array(w281) -> (w285:u16[])
                        n281 = Number To Decimal String(number=w285) -> (decimal integer string=w283:string[])  [unwired: 1 in]
                        n282 = String To Path(string="C:\\TCS\\SETUP\\INSTRUMENTOS.DAT") -> (path=w294:path)
                        n283 = Build Array(w283) -> (w284:string[][])
                        n284 = String To Path(string="C:\\TCS\\SETUP\\INSTRUM_ESCOLHIDO.DAT") -> (path=w286:path)
                        n285 = Delete(path (use dialog)=w294) -> (deleted path=w293:path)  [unwired: 4 in, 2 out]
                        n286 = Transpose 2D Array(2D array=w284) -> (transposed array=w282:string[][])
                        n287 = Delete(path (use dialog)=w286) -> (deleted path=w287:path)  [unwired: 4 in, 2 out]
                        n288 = Path To String(path=w293) -> (string=w292:string)
                        n289 = Path To String(path=w287) -> (string=w288:string)
                        n290 = call "salvaexel.vi"("appended array"=w290, "file name p/ exell"=w292) -> ()  [unwired: 1 in, 1 out]
                        n291 = call "salvaexel.vi"("appended array"=w282, "file name p/ exell"=w288) -> ()  [unwired: 1 in, 1 out]
                      }
                      frame #1 {
                        # "Valores Instrumentos Auto Guider"
                        # "Recarrega Globais necessárias"
                        n292 = local read "Tabela Instrumentos"() -> (w326:string[][])
                        n293 = Index Array(array=w326, index (col)=0 ("disabled index (col)")) -> (element=w323:string[])  [unwired: 1 in]
                        n294 = global write "Global_Telescopio.vi" "Lista Instrumentos"(w323) -> ()
                        n295 = local read "Instrumento"() -> (w322:u16)
                        n296 = property on="Instrumento" class="Ring (strict)"("Strings []"=w323) -> ()  [unwired: 2 in, 2 out]
                        n297 = global write "Global_Telescopio.vi" "Instrum"(w322) -> ()
                        n298 = Index Array(array=w326, index (row)=w322) -> (element=w324:string[])  [unwired: 1 in]
                        n299 = Index Array(array=w324, index #1=1 ("index")) -> (element #1=w318:string, element #2=w314:string, element #3=w311:string, element #4=w308:string, element #5=w304:string, element #6=w302:string, element #7=w297:string, element #8=w295:string)  [unwired: 7 in]
                        n300 = global write "Global_Telescopio.vi" "Foco Instrumento"(w295) -> ()
                        n301 = call "point_to_comma.vi"("Lat_A"=w302) -> ("Saída"=w303:string)
                        n302 = call "point_to_comma.vi"("Lat_A"=w297) -> ("Saída"=w296:string)
                        n303 = call "Comma_to_Point.vi"("Lat_A"=w318) -> ("Saída"=w319:string)
                        n304 = call "Comma_to_Point.vi"("Lat_A"=w314) -> ("Saída"=w315:string)
                        n305 = call "Comma_to_Point.vi"("Lat_A"=w304) -> ("Saída"=w305:string)
                        n306 = Fract/Exp String To Number(string=w303) -> (number=w301:dbl)  [unwired: 3 in, 1 out]
                        n307 = Fract/Exp String To Number(string=w296) -> (number=w299:dbl)  [unwired: 3 in, 1 out]
                        n308 = call <vilib>:"Trim Whitespace.vi"("string"=w311) -> ("trimmed string"=w313:string)  [unwired: 1 in]
                        n309 = call <vilib>:"Trim Whitespace.vi"("string"=w308) -> ("trimmed string"=w310:string)  [unwired: 1 in]
                        n310 = call "Arcsec to Rad.vi"("Arcsec"=w301) -> ("rad"=w300:dbl)
                        n311 = call "Arcsec to Rad.vi"("Arcsec"=w299) -> ("rad"=w298:dbl)
                        n312 = call "Formata_Numeros.vi"("Formato ex-> 7.2"="7.2", "Valor num"=w319) -> ("resulting string"=w320:string)
                        n313 = call "Formata_Numeros.vi"("Formato ex-> 7.2"="7.2", "Valor num"=w315) -> ("resulting string"=w316:string)
                        n314 = call "Formata_Numeros.vi"("Formato ex-> 7.2"="5.3", "Valor num"=w305) -> ("resulting string"=w306:string)
                        n315 = global write "Global_Telescopio.vi" "CalagemDEC_Inicial"(w297) -> ()
                        n316 = To Upper Case(1:w313) -> (0:w312:string)
                        n317 = To Upper Case(1:w310) -> (0:w309:string)
                        n318 = global write "Global_Telescopio.vi" "Calagem AH"(w300) -> ()
                        n319 = global write "Global_Telescopio.vi" "Calagem DEC"(w298) -> ()
                        n320 = global write "Global_Telescopio.vi" "CalagemAH_Inicial"(w302) -> ()
                        n321 = global write "Global_Telescopio.vi" "rotator_def"(w320) -> ()
                        n322 = global write "Global_Telescopio.vi" "guide_nor"(w316) -> ()
                        n323 = global write "Global_Telescopio.vi" "guide_esp"(w312) -> ()
                        n324 = global write "Global_Telescopio.vi" "esc_placa"(w306) -> ()
                        n325 = global write "Global_Telescopio.vi" "guide_cas"(w309) -> ()
                      }
                      frame #2 {
                        n326 = disable-structure shown="Disabled" {
                          frame Disabled {
                            # "25/10/2012 - Teste: deve ser retirado"
                            n327 = case shown="True" "Case Constant\n(See Context Help) 4" {
                              frame False {
                              }
                              frame True {
                                # "Salva as Globais Calagem"
                                n328 = global read "Global_Telescopio.vi" "Calagem AH"() -> (w332:dbl)
                                n329 = global read "Global_Telescopio.vi" "Calagem DEC"() -> (w331:dbl)
                                n330 = call "Rad to Arcsec.vi"("Radiano"=w332) -> ("Arcsec"=w329:dbl)
                                n331 = call "Rad to Arcsec.vi"("Radiano"=w331) -> ("Arcsec"=w330:dbl)
                                n332 = Build Array(w329, w330) -> (w339:dbl[])
                                n333 = Number To Fractional String(number=w339, precision (6)=i16 8) -> (F-format string=w340:string[])  [unwired: 2 in]
                                n334 = Build Array(w340) -> (w334:string[][])
                                n335 = String To Path(string="C:\\TCS\\SETUP\\GLOBAIS_CALAGEM.DAT") -> (path=w335:path)
                                n336 = Transpose 2D Array(2D array=w334) -> (transposed array=w333:string[][])
                                n337 = Delete(path (use dialog)=w335) -> (deleted path=w336:path)  [unwired: 4 in, 2 out]
                                n338 = Path To String(path=w336) -> (string=w337:string)
                                n339 = call "salvaexel.vi"("appended array"=w333, "file name p/ exell"=w337) -> ()  [unwired: 1 in, 1 out]
                              }
                            }
                          }
                          frame Enabled {
                          }
                        }
                      }
                    }
                  }
                }
              }
            }
          }
          frame "Utils" {
            n340 = stacked-sequence {
              frame #0 {
                (unwired) FALSE ("True = hora")
                n341 = global read "Global_Telescopio.vi" "Azimute GRAUS"() -> (→"Azimute":dbl)
                n342 = global read "Global_Telescopio.vi" "Zenital angle GRAUS"() -> (→"Ângulo Zenital":dbl)
                n343 = call <vilib>:"Trim Whitespace.vi"("string"="Dest Dec") -> ("trimmed string"=w349:string)  [unwired: 1 in]
                n344 = call <vilib>:"Trim Whitespace.vi"("string"="Hour Angle") -> ("trimmed string"=w346:string)  [unwired: 1 in]
                n345 = call "Comma_to_Point.vi"("Lat_A"=w349) -> ("Saída"=w348:string)
                n346 = call "Comma_to_Point.vi"("Lat_A"=w346) -> ("Saída"=w344:string)
                n347 = call "hms_rad.vi"("Texto Graus"=w348) -> ("radianos"=→"DestDEC":dbl)  [unwired: 4 in]
                n348 = call "hms_rad.vi"("True = hora"=TRUE, "Texto Graus"=w344) -> ("radianos"=→"DestAH":dbl)  [unwired: 3 in]
              }
              frame #1 {
                n349 = case shown="True" "SALVA CONFIG" {
                  frame False {
                  }
                  frame True {
                    n350 = local read "Raio Máximo"() -> (w381:dbl)
                    n351 = local read "Limite Oeste"() -> (w368:dbl)
                    n352 = local read "Limite Leste"() -> (w369:dbl)
                    n353 = local read "DestAH"() -> (w387:dbl)
                    n354 = local read "DestCUP"() -> (w388:i32)
                    n355 = local read "Z_Segurança"() -> (w384:dbl)
                    n356 = local read "Z_Libera"() -> (w383:dbl)
                    n357 = local read "DestDEC"() -> (w386:dbl)
                    n358 = local read "Z_Max"() -> (w382:dbl)
                    n359 = global write "Global_Telescopio.vi" "Raio Máximo"(w381) -> ()
                    n360 = global write "Global_Telescopio.vi" "Limite EAST"(w369) -> ()
                    n361 = global write "Global_Telescopio.vi" "Limite WEST"(w368) -> ()
                    n362 = global write "Global_Telescopio.vi" "DestAH"(w387) -> ()
                    n363 = global write "Global_Telescopio.vi" "DestDEC"(w386) -> ()
                    n364 = global write "Global_Telescopio.vi" "DestCUP"(w388) -> ()
                    n365 = local read "Tempo delay"() -> (w367:i32)
                    n366 = global write "Global_Telescopio.vi" "Tempo delay"(w367) -> ()
                    n367 = local read "Hora vent inicial"() -> (w358:i32)
                    n368 = local read "Tempo Atualização All Sky"() -> (w370:i32)
                    n369 = local read "Tempo Atualização Cam 0"() -> (w371:i32)
                    n370 = local read "Tempo Atualização Cam 1"() -> (w372:i32)
                    n371 = local read "Tempo Atualização Cam 2"() -> (w373:i32)
                    n372 = local read "Tempo Atualização Cam 3"() -> (w374:i32)
                    n373 = global write "Global_Telescopio.vi" "Tempo Atulização Cam 0"(w371) -> ()
                    n374 = global write "Global_Telescopio.vi" "Tempo Atulização Cam 1"(w372) -> ()
                    n375 = global write "Global_Telescopio.vi" "Tempo Atulização Cam 2"(w373) -> ()
                    n376 = global write "Global_Telescopio.vi" "Tempo Atulização Cam 3"(w374) -> ()
                    n377 = global write "Global_Telescopio.vi" "Tempo Atulização All Sky"(w370) -> ()
                    n378 = local read "Hora vent final"() -> (w357:i32)
                    n379 = Number To Decimal String(number=w358) -> (decimal integer string=w356:string)  [unwired: 1 in]
                    n380 = Number To Decimal String(number=w357) -> (decimal integer string=w355:string)  [unwired: 1 in]
                    n381 = local read "habilita supervisao"() -> (w366:bool)
                    n382 = global write "Global_Telescopio.vi" "Habilita supervisao"(w366) -> ()
                    n383 = global write "Global_Telescopio.vi" "Hora vent inicial"(w356) -> ()
                    n384 = local read "Enable ventilador"() -> (w363:bool)
                    n385 = global write "Global_Telescopio.vi" "Enable ventilador"(w363) -> ()
                    n386 = global write "Global_Telescopio.vi" "Hora vent final"(w355) -> ()
                    n387 = local read "Caminho camera"() -> (w359:string)
                    n388 = global write "Global_Telescopio.vi" "Caminho camera"(w359) -> ()
                    n389 = case shown="True" w366 {
                      tunnel: [0 1] -> w365
                      frame False {
                      }
                      frame True {
                      }
                    }
                    n390 = case shown="True" w363 {
                      tunnel: [0 1] -> w364
                      frame False {
                      }
                      frame True {
                      }
                    }
                    n391 = Build Array(w387, w386, w388, w384, w383, w382, w381, w369, w368, w370, w371, w372, w373, w374, w367, w365, w364) -> (w393:dbl[])
                    n392 = Number To Fractional String(number=w393, precision (6)=i16 8) -> (F-format string=w361:string[])  [unwired: 2 in]
                    n393 = String To Path(string="C:\\TCS\\SETUP\\Utils.txt") -> (path=w391:path)
                    n394 = local read "Tabela Proteção"() -> (w375:string[][])
                    n395 = String To Path(string="C:\\TCS\\SETUP\\TABELA_PROTE敲O.DAT") -> (path=w378:path)
                    n396 = Delete(path (use dialog)=w378) -> (deleted path=w379:path)  [unwired: 4 in, 2 out]
                    n397 = global write "Global_Telescopio.vi" "Tabela Proteção"(w375) -> ()
                    n398 = Delete(path (use dialog)=w391) -> (deleted path=w390:path)  [unwired: 4 in, 2 out]
                    n399 = Path To String(path=w379) -> (string=w380:string)
                    n400 = Transpose 2D Array(2D array=w375) -> (transposed array=w377:string[][])
                    n401 = Path To String(path=w390) -> (string=w389:string)
                    n402 = local read "Senha LEAF"() -> (w354:string)
                    n403 = Build Array (concatenate)(w361, w359, w356, w355, w354) -> (w360:string[])
                    n404 = Build Array(w360) -> (w362:string[][])
                    n405 = Transpose 2D Array(2D array=w362) -> (transposed array=w392:string[][])
                    n406 = global write "Global_Telescopio.vi" "Senha LEAF"(w354) -> ()
                    n407 = call "salvaexel.vi"("appended array"=w377, "file name p/ exell"=w380) -> ()  [unwired: 1 in, 1 out]
                    n408 = call "salvaexel.vi"("appended array"=w392, "file name p/ exell"=w389) -> ()  [unwired: 1 in, 1 out]
                  }
                }
              }
              frame #2 {
                n409 = case shown="True" "Download_Finals2000A.all" {
                  selector: "Download_Finals2000A.all" -> [w401 w404]
                  tunnel: [w401 FALSE] -> w399
                  frame False {
                  }
                  frame True {
                    n410 = flat-sequence {
                      tunnel: w404 -> [w406]
                      tunnel: [w406] -> w402
                      tunnel: w402 -> [w409]
                      frame #0 {
                        n411 = local write "DownloadOK"(FALSE) -> ()
                      }
                      frame #1 {
                        (unwired) "http://maia.usno.navy.mil/ser7/finals2000A.all" ("URL")
                        (unwired) "http://toshi.nofs.navy.mil/ser7/finals2000A.all" ("URL")
                        # "http://maia.usno.navy.mil/ser7/finals2000A.all\nna pasta C:\\TCS\\ARQUIVOS\\"
                        n412 = local write "DownloadWait"(w409) -> ()
                        n413 = property on="DownloadWait" class="Bool (strict)"("Blinking"=w409) -> ()  [unwired: 2 in, 2 out]
                        n414 = property on="DownloadWait" class="Bool (strict)"("Visible"=w409) -> ()  [unwired: 2 in, 2 out]
                        n415 = String To Path(string="C:\\TCS\\ARQUIVOS\\finals2000A.all" ("URL")) -> (path=w411:path)
                        n416 = call "URL Get Document.vi"("file path (NAP)"=w411, "URL"="URL do finals2000A.all:") -> ("success"=→"DownloadOK":bool)  [unwired: 5 in, 4 out]
                      }
                    }
                  }
                }
                "DownloadWait" <- w399
                n417 = property on="DownloadWait" class="Bool (strict)"("Blinking"=w399) -> ()  [unwired: 2 in, 2 out]
                n418 = property on="DownloadWait" class="Bool (strict)"("Visible"=w399) -> ()  [unwired: 2 in, 2 out]
              }
            }
          }
        }
        n419 = Wait Until Next ms Multiple(millisecond multiple=u32 200) -> ()  [unwired: 1 out]
      }
    }
    frame #2 {
    }
  }
